vi "Test.vi"   [LabVIEW 2015, in "ConfigHelper.lvlib"]
uses:
  ConfigHelper.lvlib
  <vilib>/addons/PointValueMap/PointValueMap.lvlib
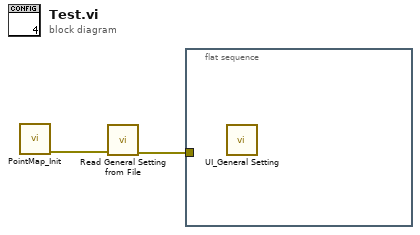
[diagram p0: block diagram]
diagram:
  n1 = call <vilib>:"PointMap_Init.vi"() -> ("error out"=w2:errorcluster)  [unwired: 11 in]
  n2 = call "Read General Setting from File.vi"("error in (no error)"=w2) -> ("error out"=w1:errorcluster)  [unwired: 10 in]
  n3 = flat-sequence {
    tunnel: w1 -> [_]
    frame #0 {
      n4 = call "UI_General Setting.vi"() -> ()  [unwired: 11 in, 1 out]
    }
  }
